vi "Configure Trigger (External).vi"(0 "VISA resource name":refnum<visa-resource-name>, 5 "Trigger Level (0 V)":dbl, 7 "Attenuation Factor (10)":dbl=10.0, 11 "error in (no error)":errorcluster) -> (4 "VISA resource name out":refnum<visa-resource-name>, 15 "error out":errorcluster)   [LabVIEW 2009, in "Tektronix DPO MSO 2000 4000 Series.lvlib"]
doc: "Configures the trigger level for the auxiliary port and attenuation factor value of the external probe connector."
uses:
  <instrlib>/Tektronix DPO MSO 2000 4000 Series/Tektronix DPO MSO 2000 4000 Series.lvlib
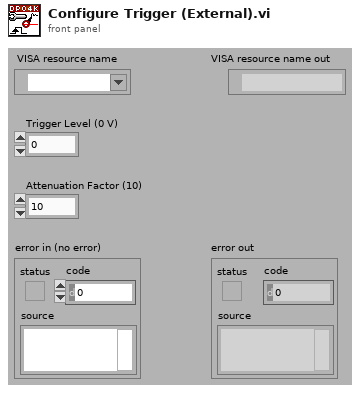
[diagram p1: front panel]
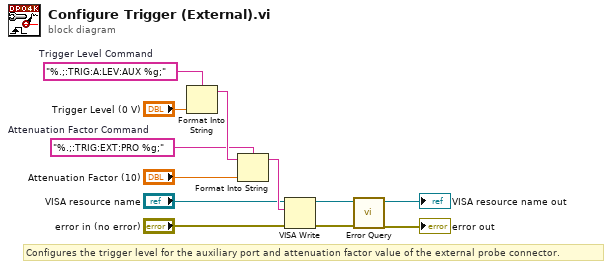
[diagram p0: block diagram]
diagram:
  w9 = "%.;:TRIG:EXT:PRO %g;"  # Attenuation Factor Command
  w12 = "%.;:TRIG:A:LEV:AUX %g;"  # Trigger Level Command
  # "Configures the trigger level for the auxiliary port and attenuation factor value of the external probe connector."
  n1 = Format Into String(format string=w12, "Trigger Level (0 V)") -> (resulting string=w10:string)  [unwired: 2 in, 1 out]
  n2 = Format Into String(format string=w9, initial string=w10, "Attenuation Factor (10)") -> (resulting string=w7:string)  [unwired: 1 in, 1 out]
  n3 = VISA Write(VISA resource name="VISA resource name", write buffer=w7, error in (no error)="error in (no error)") -> (VISA resource name out=w4:refnum<visa-resource-name>, error out=w3:errorcluster)  [unwired: 1 out]
  n4 = call <instrlib>:"Error Query.vi"("error in (no error)"=w3, "VISA resource name"=w4) -> ("error out"=→"error out":errorcluster, "VISA resource name out"=→"VISA resource name out":refnum<visa-resource-name>)  [unwired: 6 in, 2 out]
